vi "Squareness_2.vi"() -> ()   [LabVIEW 2020]
uses:
  Support/Controls/Cmd_Mouse Popup.ctl
  Support/Controls/Clst_Initialize Input.ctl
  Support/Controls/Cmd_Var Data IO.ctl
  Support/Controls/Cmd_STD select.ctl
  Variables/Global_Cal Info.vi
  Variables/Global_Cal STD.vi
  <vilib>/express/express arith-compare/Formula/XNode/ExpressFormulaBlockNode.xnode
panel:
  out "기준기분해능 (μm)":string
  in  "기준기 설정":string(combo)
  out "직각도":string[][](table) caption="직각도 (μm/m)"
  out "단위":string
  out "최고점":string
  out "최저점":string
  in  "Spec 변경":bool
  in  "Random":bool
  out "Spec":string[][](table)
  out "제목":string
  out "에러 출력":errorcluster
  out "Condition":string[][](table) caption="2. 직선성 시험"
  in  "Measured":string[][](table) caption="기준기 지시값 (μm)"
  out "Load?":bool
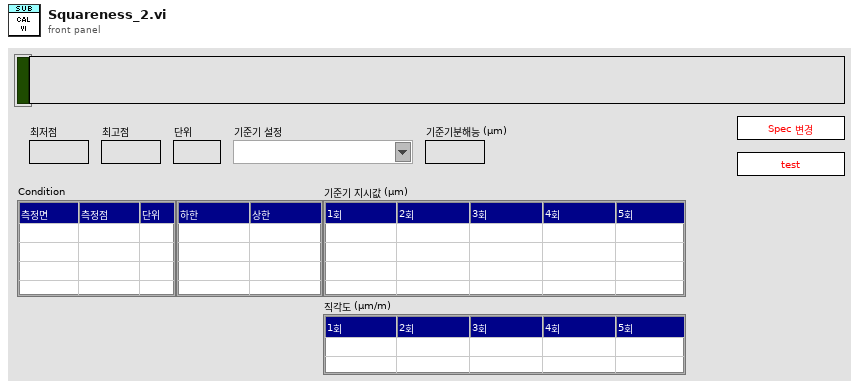
[diagram p1: front panel]
types:
  T1 = typedef "Cmd_Mouse Popup.ctl" = enum16{"활성화", "메뉴선택"}
  T2 = cluster{"Shift":bool, "Ctrl":bool, "Alt":bool, "Cmd":bool, "Opt":bool}
  T3 = typedef "Clst_Initialize Input.ctl" = cluster{"Initialize 1":cluster{"Condition":refnum<vi>[], "Spec":refnum<vi>[], "Measured":refnum<vi>[], "Resolution":refnum<vi>[], "Func_ext":string, "제목":refnum<vi>, "Measured_ADJ":refnum<vi>[]}, "Initialize 2":cluster{"문자열":refnum<vi>[], "콤보박스":refnum<vi>[], "링":refnum<vi>[], "열거형":refnum<vi>[], "테이블":refnum<vi>[], "여러열":refnum<vi>[], "디지털(DBL)":refnum<vi>[], "3D string":refnum<vi>[], "ctrl":refnum<vi>[], "boolean":refnum<vi>[]}}
  T4 = typedef "Cmd_Var Data IO.ctl" = enum16{"Condition", "Condition Default", "Condition_Temp", "Resolution", "Resolution Default", "Resolution Old", "Spec", "Spec Default", "Spec Old", "Spec Temp", "Result", "Result2", "Result3", "Result_Temp", "Result_ADJ", "Result_ADJ2", "STD1", "STD2", "STD3", "STD4", "STD5", "STD Temp", "CMC", "CMC Default"}
  T5 = typedef "Cmd_STD select.ctl" = enum16{"기본", "DMM", "Electronic Micrometer", "Fine Angle Generator", "Measuring Projector", "Precision Square", "Power Supply", "Ring Gauge", "Straight Edge", "Thermo-Hygrometer", "Calibrator"}
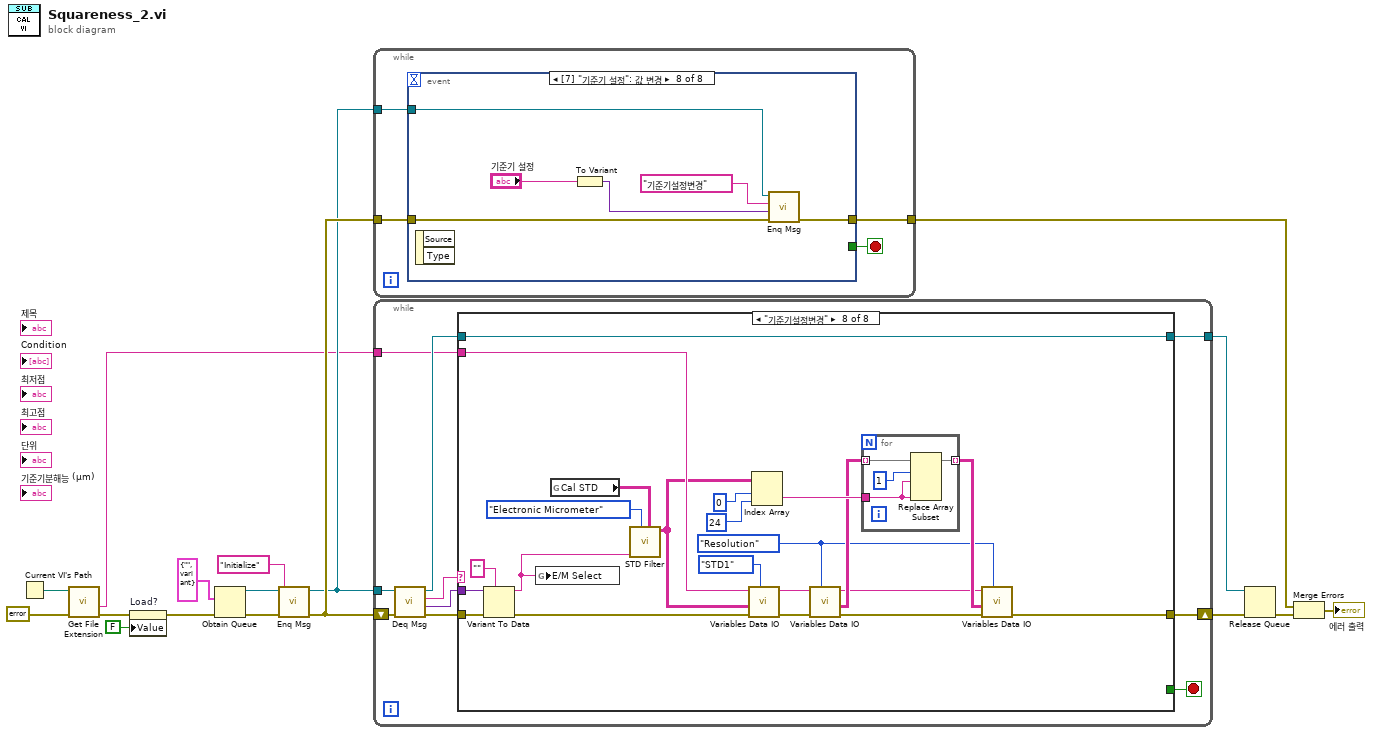
[diagram p0: block diagram]
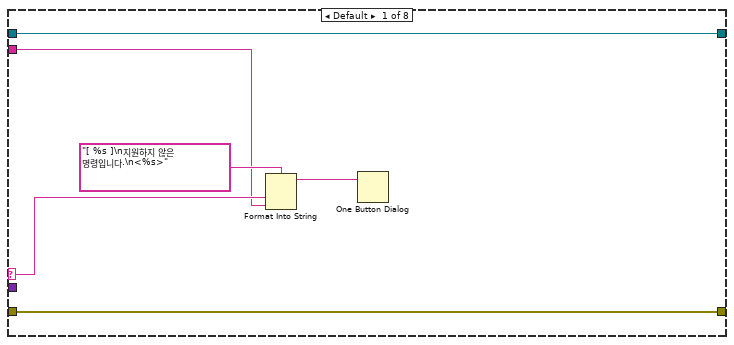
[diagram p2: hidden frame]
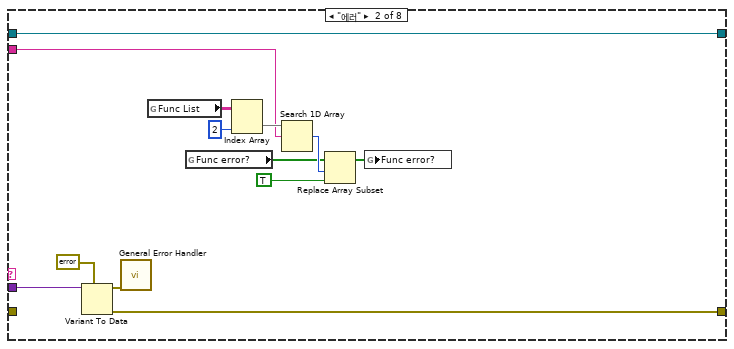
[diagram p3: hidden frame]
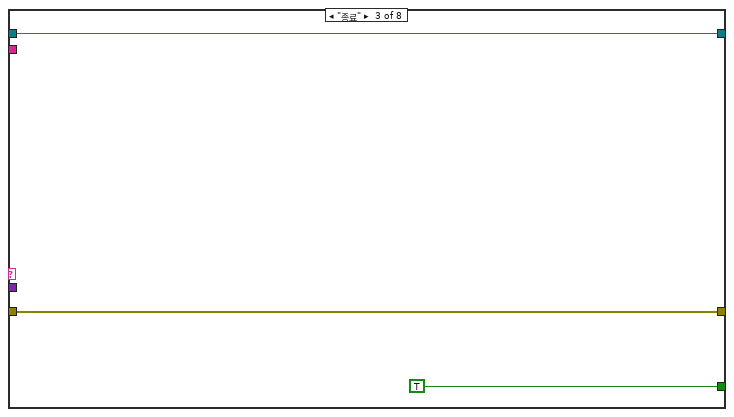
[diagram p4: hidden frame]
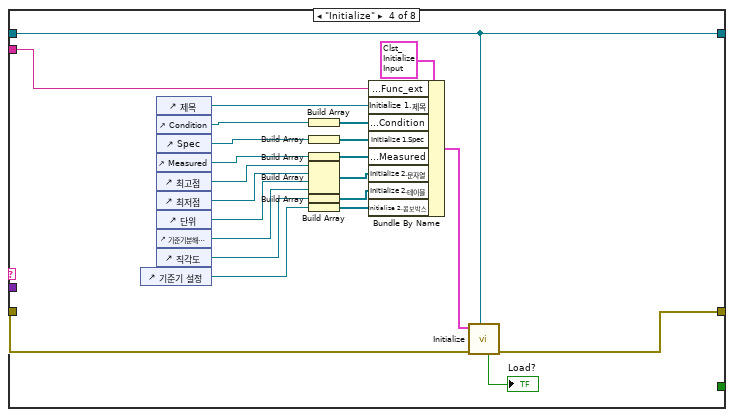
[diagram p5: hidden frame]
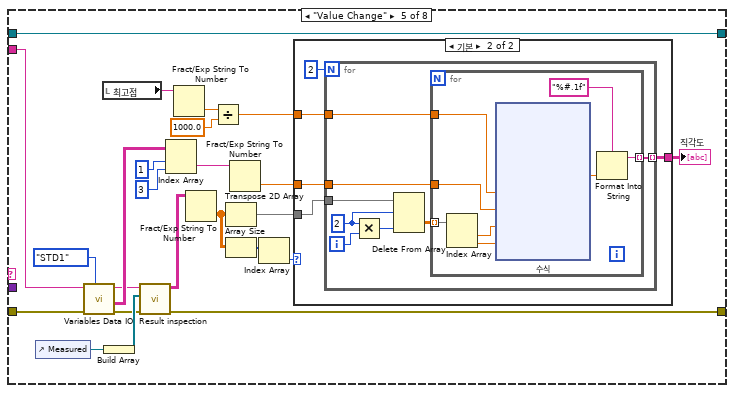
[diagram p6: hidden frame]
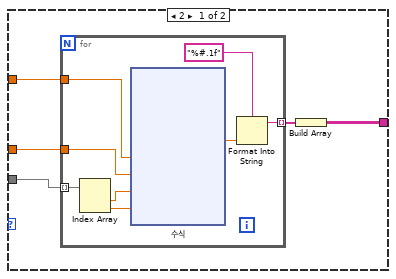
[diagram p7: hidden frame]
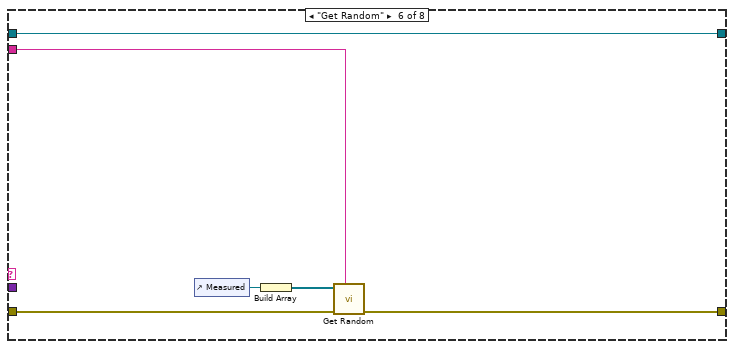
[diagram p8: hidden frame]
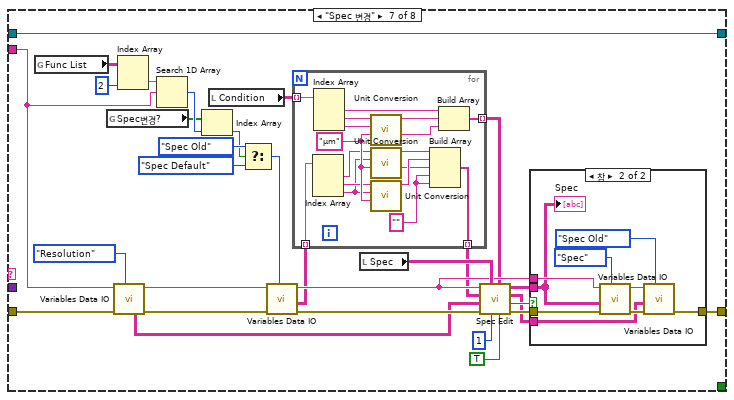
[diagram p9: hidden frame]
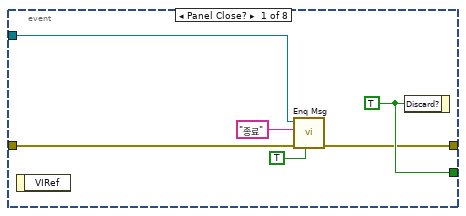
[diagram p11: hidden frame]
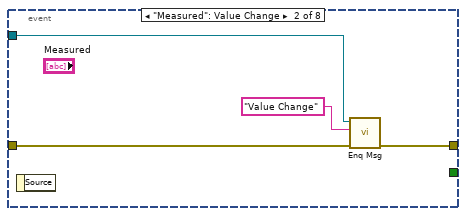
[diagram p12: hidden frame]
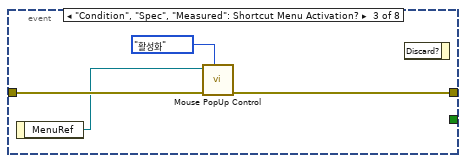
[diagram p13: hidden frame]
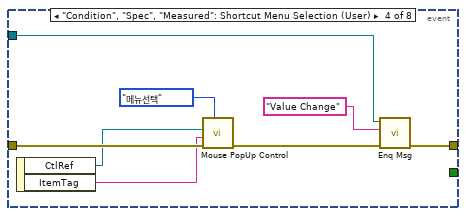
[diagram p14: hidden frame]
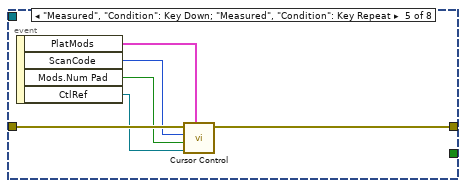
[diagram p15: hidden frame]
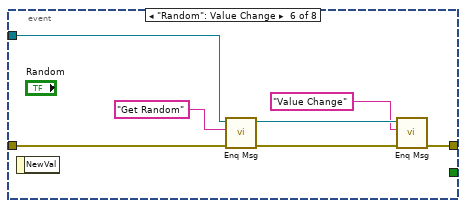
[diagram p16: hidden frame]
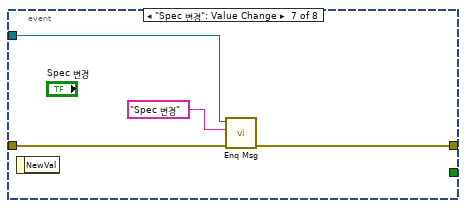
[diagram p17: hidden frame]
diagram:
  n1 = Current VI's Path() -> (path=w5:path)
  n2 = call <vilib>:"Get File Extension.vi"("error in (no error)"=errorcluster {"status"=FALSE, "code"=0, "source"=""} ("에러 상수"), "file"=w5) -> ("error out"=w3:errorcluster, "filename without extension"=w4:string)  [unwired: 5 in, 3 out]
  n3 = property on="Load?" class="Bool (엄격한)"(error in=w3, "Value"=FALSE ("Load?")) -> (error out=w2:errorcluster)  [unwired: 1 in, 1 out]
  n4 = Obtain Queue(element data type=cluster{"메세지":string, "값":variant} {"메세지"="", "값"=variant} ("Message Cluster"), error in (no error)=w2) -> (queue out=w14:refnum<queue>, error out=w16:errorcluster)  [unwired: 3 in, 1 out]
  n5 = call "Enq Msg.vi"("에러 입력(에러 없음)"=w16, "메세지"="Initialize", "큐 입력"=w14) -> ("에러 출력"=w15:errorcluster, "큐 출력"=w12:refnum<queue>)  [unwired: 7 in]
  n6 = while {
    tunnel: w15 -> [w19]
    tunnel: w12 -> [w20]
    tunnel: [w18] -> w9
    stop <- w21 stop-if-true
    n7 = event shown="[7] \"기준기 설정\": 값 변경" {
      selector: _ -> [_ _ _ _ _ _ _ _]
      dyn-events: _ -> [_ _ _ _ _ _ _ _]
      timeout: _ -> [_ _ _ _ _ _ _ _]
      tunnel: [w27 _ _ _ _ _ _ _] -> w21
      tunnel: w20 -> [w25 w31 _ w36 _ w54 w58 w64]
      tunnel: w19 -> [w26 w29 w35 w43 w49 w55 w59 w65]
      tunnel: [w23 w30 w34 w37 w48 w50 w57 w63] -> w18
      event Panel Close? {
        w27 = TRUE ("버림?")
        n8 = event-data() -> ()  [unwired: 1 in, 1 out]
        n9 = call "Enq Msg.vi"("우선순위 메시지?"=TRUE, "에러 입력(에러 없음)"=w26, "메세지"="종료", "큐 입력"=w25) -> ("에러 출력"=w23:errorcluster)  [unwired: 6 in, 1 out]
        n10 = event-data("Discard?"=w27) -> ()  [unwired: 1 in, 1 out]
      }
      event "Measured": Value Change {
        n11 = event-data() -> ()  [unwired: 1 in, 1 out]
        n12 = call "Enq Msg.vi"("에러 입력(에러 없음)"=w29, "메세지"="Value Change", "큐 입력"=w31) -> ("에러 출력"=w30:errorcluster)  [unwired: 7 in, 1 out]
      }
      event "Condition", "Spec", "Measured": Shortcut Menu Activation? {
        n13 = event-data() -> ("MenuRef"=w33:refnum<k9>)  [unwired: 1 in]
        n14 = call "Mouse PopUp Control.vi"("type"=Cmd_Mouse_Popup."활성화", "error in"=w35, "메뉴 참조"=w33) -> ("error out"=w34:errorcluster)  [unwired: 8 in]
        n15 = event-data() -> ()  [unwired: 2 in, 1 out]
      }
      event "Condition", "Spec", "Measured": Shortcut Menu Selection (User) {
        n16 = event-data() -> ("CtlRef"=w41:refnum<vi>, "ItemTag"=w40:string)  [unwired: 1 in]
        n17 = call "Mouse PopUp Control.vi"("type"=Cmd_Mouse_Popup."메뉴선택", "error in"=w43, "아이템 태그"=w40, "Tbl 참조 번호"=w41) -> ("error out"=w38:errorcluster)  [unwired: 7 in]
        n18 = call "Enq Msg.vi"("에러 입력(에러 없음)"=w38, "메세지"="Value Change", "큐 입력"=w36) -> ("에러 출력"=w37:errorcluster)  [unwired: 7 in, 1 out]
      }
      event "Measured", "Condition": Key Down; "Measured", "Condition": Key Repeat {
        n19 = event-data() -> ("PlatMods"=w44:T2, "ScanCode"=w47:i16, "Mods.Num Pad"=w46:bool, "CtlRef"=w45:refnum<vi>)  [unwired: 1 in]
        n20 = call "Cursor Control.vi"("플랫폼 조합키"=w44, "참조"=w45, "Num Pad"=w46, "ScanCode"=w47, "error in"=w49) -> ("error out"=w48:errorcluster)  [unwired: 5 in, 1 out]
      }
      event "Random": Value Change {
        n21 = event-data() -> ()  [unwired: 1 in, 1 out]
        n22 = call "Enq Msg.vi"("에러 입력(에러 없음)"=w55, "메세지"="Get Random", "큐 입력"=w54) -> ("에러 출력"=w53:errorcluster, "큐 출력"=w52:refnum<queue>)  [unwired: 7 in]
        n23 = call "Enq Msg.vi"("에러 입력(에러 없음)"=w53, "메세지"="Value Change", "큐 입력"=w52) -> ("에러 출력"=w50:errorcluster)  [unwired: 7 in, 1 out]
      }
      event "Spec 변경": Value Change {
        n24 = event-data() -> ()  [unwired: 1 in, 1 out]
        n25 = call "Enq Msg.vi"("에러 입력(에러 없음)"=w59, "메세지"="Spec 변경", "큐 입력"=w58) -> ("에러 출력"=w57:errorcluster)  [unwired: 7 in, 1 out]
      }
      event "기준기 설정": Value Change {
        n26 = event-data() -> ()  [unwired: 1 in, 2 out]
        n27 = To Variant(anything="기준기 설정") -> (Variant=w61:variant)
        n28 = call "Enq Msg.vi"("에러 입력(에러 없음)"=w65, "값"=w61, "메세지"="기준기설정변경", "큐 입력"=w64) -> ("에러 출력"=w63:errorcluster)  [unwired: 6 in, 1 out]
      }
    }
  }
  n29 = while {
    shift-right: [w76] -> w11
    shift-left: w15 -> [w75]
    tunnel: w12 -> [w73]
    tunnel: [w68] -> w10
    tunnel: w4 -> [w67]
    stop <- w69 stop-if-true
    n30 = call "Deq Msg.vi"("에러 입력(에러 없음)"=w75, "큐 입력"=w73) -> ("에러 출력"=w74:errorcluster, "값"=w70:variant, "메세지"=w72:string, "큐 출력"=w71:refnum<queue>)  [unwired: 6 in]
    n31 = case shown="\"기준기설정변경\"" w72 {
      selector: w72 -> [w78 _ _ _ _ _ _ _]
      tunnel: w74 -> [w82 _ w98 w121 w128 w209 w236 w285]
      tunnel: [w82 w92 w98 w108 w125 w210 w239 w271] -> w76
      tunnel: w71 -> [w81 w91 w96 w109 w145 w213 w243 w292]
      tunnel: w70 -> [_ w93 _ _ _ _ _ w284]
      tunnel: [_ _ TRUE ("버림?") _ _ _ _ _] -> w69
      tunnel: [w81 w91 w96 w109 w145 w213 w243 w292] -> w68
      tunnel: w67 -> [w77 w83 _ w110 w136 w208 w223 w283]
      frame Default {
        n32 = Format Into String(format string="[ %s ]\n지원하지 않은 명령입니다.\n<%s>" ("메시지"), w78, w77) -> (resulting string=w79:string)  [unwired: 2 in, 1 out]
        n33 = One Button Dialog(message=w79) -> ()  [unwired: 1 in, 1 out]
      }
      frame "에러" {
        n34 = Variant To Data(type=errorcluster {"status"=FALSE, "code"=0, "source"=""} ("에러 출력"), Variant=w93) -> (data=w95:errorcluster, error out=w92:errorcluster)  [unwired: 1 in]
        n35 = call <vilib>:"General Error Handler.vi"("error in (no error)"=w95) -> ()  [unwired: 10 in, 5 out]
        n36 = global read "Global_Cal Info.vi" "Func List"() -> (w85:string[][])
        n37 = global read "Global_Cal Info.vi" "Func error?"() -> (w88:bool[])
        n38 = Index Array(array=w85, index (col)=2 ("비활성화된 인덱스 (열)")) -> (element=w86:string[])  [unwired: 1 in]
        n39 = Search 1D Array(1D array=w86, element=w83) -> (index of element=w89:i32)  [unwired: 1 in]
        n40 = Replace Array Subset(array=w88, new element=TRUE ("새 원소/부분배열"), index=w89) -> (w90:bool[])
        n41 = global write "Global_Cal Info.vi" "Func error?"(w90) -> ()
      }
      frame "종료" {
      }
      frame "Initialize" {
        n42 = control-ref of="기준기 설정"() -> (w100:refnum<vi>)
        n43 = control-ref of="제목"() -> (w113:refnum<vi>)
        n44 = control-ref of="Condition"() -> (w118:refnum<vi>)
        n45 = control-ref of="Spec"() -> (w112:refnum<vi>)
        n46 = control-ref of="Measured"() -> (w115:refnum<vi>)
        n47 = control-ref of="최고점"() -> (w106:refnum<vi>)
        n48 = control-ref of="최저점"() -> (w105:refnum<vi>)
        n49 = control-ref of="단위"() -> (w104:refnum<vi>)
        n50 = control-ref of="기준기분해능 (μm)"() -> (w99:refnum<vi>)
        n51 = control-ref of="직각도"() -> (w103:refnum<vi>)
        n52 = Build Array(w118) -> (w117:refnum<vi>[])
        n53 = Build Array(w112) -> (w111:refnum<vi>[])
        n54 = Build Array(w115) -> (w116:refnum<vi>[])
        n55 = Build Array(w106, w105, w104, w99) -> (w114:refnum<vi>[])
        n56 = Build Array(w103) -> (w102:refnum<vi>[])
        n57 = Build Array(w100) -> (w101:refnum<vi>[])
        n58 = Bundle By Name(cluster=T3 {"Initialize 1"={"Condition"=[], "Spec"=[], "Measured"=[], "Resolution"=[], "Func_ext"="", "제목"=refnum, "Measured_ADJ"=[]}, "Initialize 2"={"문자열"=[], "콤보박스"=[], "링"=[], "열거형"=[], "테이블"=[], "여러열"=[], "디지털(DBL)"=[], "3D string"=[], "ctrl"=[], "boolean"=[]}} ("입력 클러스터"), "Initialize 1.Func_ext"=w110, "Initialize 1.제목"=w113, "Initialize 1.Condition"=w117, "Initialize 1.Spec"=w111, "Initialize 1.Measured"=w116, "Initialize 2.문자열"=w114, "Initialize 2.테이블"=w102, "Initialize 2.콤보박스"=w101) -> (w119:T3)
        n59 = call "Initialize.vi"("큐 입력"=w109, "error in"=w121, "입력 클러스터"=w119) -> ("error out"=w108:errorcluster, "Load?"=→"Load?":bool)  [unwired: 5 in, 2 out]
      }
      frame "Value Change" {
        n60 = control-ref of="Measured"() -> (w144:refnum<vi>)
        n61 = call "Variables Data IO.vi"("Select"=Cmd_Var_Data_IO."STD1", "error in"=w128, "Func_ext"=w136) -> ("error out"=w126:errorcluster, "Data Out"=w134:string[][], "Func_ext Out"=w127:string)  [unwired: 6 in]
        n62 = local read "최고점"() -> (w140:string)
        n63 = Build Array(w144) -> (w143:refnum<vi>[])
        n64 = call "Result inspection.vi"("error in"=w126, "Ref. Data (Inspection)"=w143, "Func ext"=w127) -> ("error out"=w125:errorcluster, "Data (spec 적용)"=w142:string[][])  [unwired: 5 in, 2 out]
        n65 = Index Array(array=w134, index (row)=1 ("인덱스 (행)"), index (col)=3 ("비활성화된 인덱스 (열)")) -> (element=w131:string)
        n66 = Fract/Exp String To Number(string=w140) -> (number=w139:dbl)  [unwired: 3 in, 1 out]
        n67 = Fract/Exp String To Number(string=w142) -> (number=w124:dbl[][])  [unwired: 3 in, 1 out]
        n68 = Divide(x=w139, y=1000.0) -> (x/y=w137:dbl)
        n69 = Transpose 2D Array(2D array=w124) -> (transposed array=w141:dbl[][])
        n70 = Array Size(array=w124) -> (size(s)=w123:i32[])
        n71 = Fract/Exp String To Number(string=w131) -> (number=w130:dbl)  [unwired: 3 in, 1 out]
        n72 = Index Array(array=w123) -> (element=w122:i32)  [unwired: 1 in]
        n73 = case shown="기본" w122 {
          tunnel: w141 -> [w150 w177]
          tunnel: w137 -> [w149 w176]
          tunnel: w130 -> [w148 w175]
          tunnel: [w146 w173] -> w129
          frame 2 {
            n74 = for {
              tunnel: w150 -> [w158] mode=indexing
              tunnel: w149 -> [w157]
              tunnel: w148 -> [w151]
              tunnel: [w152] -> w147 mode=indexing
              n75 = Index Array(array=w158) -> (element #1=w156:dbl, element #2=w155:dbl)  [unwired: 2 in]
              n76 = xnode "수식"("l"=w157, "T"=w151, "dmin"=w156, "dmax"=w155) -> ("결과"=w154:dbl)  [unwired: 1 in, 1 out]
              n77 = Format Into String(format string="%#.1f" ("포맷 문자열"), w154) -> (resulting string=w152:string)  [unwired: 2 in, 1 out]
            }
            n78 = Build Array(w147) -> (w146:string[][])
          }
          frame Default {
            n79 = for {
              N: 2 -> [_]
              tunnel: w177 -> [w182]
              tunnel: w176 -> [w185]
              tunnel: w175 -> [w184]
              tunnel: [w183] -> w173 mode=indexing
              i -> [w181]
              w180 = 2 ("길이")
              n80 = Multiply(x=w180, y=w181) -> (x*y=w179:i32)
              n81 = Delete From Array(array=w182, length=w180, index (col)=w179) -> (deleted portion=w178:dbl[][])  [unwired: 1 in, 1 out]
              n82 = for {
                tunnel: w178 -> [w193] mode=indexing
                tunnel: w185 -> [w192]
                tunnel: w184 -> [w186]
                tunnel: [w187] -> w183 mode=indexing
                n83 = Index Array(array=w193) -> (element #1=w191:dbl, element #2=w190:dbl)  [unwired: 2 in]
                n84 = xnode "수식"("l"=w192, "T"=w186, "dmin"=w191, "dmax"=w190) -> ("결과"=w189:dbl)  [unwired: 1 in, 1 out]
                n85 = Format Into String(format string="%#.1f" ("포맷 문자열"), w189) -> (resulting string=w187:string)  [unwired: 2 in, 1 out]
              }
            }
          }
        }
        "직각도" <- w129
      }
      frame "Get Random" {
        n86 = control-ref of="Measured"() -> (w212:refnum<vi>)
        n87 = Build Array(w212) -> (w211:refnum<vi>[])
        n88 = call "Get Random.vi"("Func_Ext"=w208, "에러 입력"=w209, "Meas"=w211) -> ("에러 출력"=w210:errorcluster)  [unwired: 7 in, 1 out]
      }
      frame "Spec 변경" {
        n89 = global read "Global_Cal Info.vi" "Func List"() -> (w228:string[][])
        n90 = global read "Global_Cal Info.vi" "Spec변경?"() -> (w224:bool[])
        n91 = call "Variables Data IO.vi"("Select"=Cmd_Var_Data_IO."Resolution", "error in"=w236, "Func_ext"=w223) -> ("error out"=w221:errorcluster, "Data Out"=w219:string[][], "Func_ext Out"=w220:string)  [unwired: 6 in]
        n92 = Index Array(array=w228, index (col)=2 ("비활성화된 인덱스 (열)")) -> (element=w226:string[])  [unwired: 1 in]
        n93 = Search 1D Array(1D array=w226, element=w223) -> (index of element=w225:i32)  [unwired: 1 in]
        n94 = Index Array(array=w224, index=w225) -> (element=w229:bool)
        n95 = local read "Condition"() -> (w217:string[][])
        n96 = Select(t=Cmd_Var_Data_IO."Spec Old" ("Select"), s=w229, f=Cmd_Var_Data_IO."Spec Default" ("Select")) -> (s? t:f=w222:T4)
        n97 = call "Variables Data IO.vi"("Select"=w222, "error in"=w221, "Func_ext"=w220) -> ("error out"=w238:errorcluster, "Data Out"=w215:string[][], "Func_ext Out"=w232:string)  [unwired: 6 in]
        n98 = for {
          tunnel: w217 -> [w247] mode=indexing
          tunnel: [w248] -> w216 mode=indexing
          tunnel: w215 -> [w257] mode=indexing
          tunnel: [w250] -> w214 mode=indexing
          w249 = "" ("원소")
          w258 = "μm" ("환산단위")
          n99 = Index Array(array=w257) -> (element #1=w256:string, element #2=w255:string, element #3=w254:string)  [unwired: 3 in]
          n100 = Index Array(array=w247) -> (element #1=w246:string, element #2=w260:string, element #3=w259:string)  [unwired: 3 in]
          n101 = call "Unit Conversion.vi"("환산단위"=w258, "입력단위"=w259, "입력값"=w260) -> ("환산단위"=w244:string, "환산값 (string)"=w245:string)  [unwired: 3 in, 4 out]
          n102 = call "Unit Conversion.vi"("환산단위"=w258, "입력단위"=w254, "입력값"=w256) -> ("환산단위"=w251:string, "환산값 (string)"=w253:string)  [unwired: 3 in, 4 out]
          n103 = call "Unit Conversion.vi"("환산단위"=w258, "입력단위"=w254, "입력값"=w255) -> ("환산값 (string)"=w252:string)  [unwired: 3 in, 5 out]
          n104 = Build Array(w253, w252, w251, w249, w249) -> (w250:string[])
          n105 = Build Array(w246, w245, w244) -> (w248:string[])
        }
        n106 = local read "Spec"() -> (w233:string[][])
        n107 = call "Spec Edit.vi"("0기준?"=TRUE, "Condition"=w216, "열번호(기준값)"=1, "Spec Value"=w233, "에러 입력(에러 없음)"=w238, "Resolution"=w219, "Spec Default"=w214, "Func_ext"=w232) -> ("에러 출력"=w240:errorcluster, "변경?"=w241:bool, "Spec Default out"=w235:string[][], "Spec 출력"=w242:string[][])
        n108 = case shown="참" w241 {
          tunnel: w242 -> [_ w267]
          tunnel: w240 -> [w261 w270]
          tunnel: [w261 w265] -> w239
          tunnel: w232 -> [_ w268]
          tunnel: w235 -> [_ w263]
          frame False {
          }
          frame True {
            n109 = call "Variables Data IO.vi"("Select"=Cmd_Var_Data_IO."Spec", "error in"=w270, "Data In"=w267, "Func_ext"=w268) -> ("error out"=w266:errorcluster, "Func_ext Out"=w264:string)  [unwired: 5 in, 1 out]
            n110 = call "Variables Data IO.vi"("Select"=Cmd_Var_Data_IO."Spec Old", "error in"=w266, "Data In"=w263, "Func_ext"=w264) -> ("error out"=w265:errorcluster)  [unwired: 5 in, 2 out]
            "Spec" <- w267
          }
        }
      }
      frame "기준기설정변경" {
        w277 = Cmd_Var_Data_IO."Resolution" ("Select")
        n111 = Variant To Data(error in=w285, type="", Variant=w284) -> (data=w289:string, error out=w290:errorcluster)
        n112 = global write "Global_Cal STD.vi" "E/M Select"(w289) -> ()
        n113 = global read "Global_Cal STD.vi" "Cal STD"() -> (w288:string[][])
        n114 = call "STD Filter.vi"("Cal STD in"=w288, "STD select"=Cmd_STD_select."Electronic Micrometer", "문자열(option, STD)"=w289) -> ("DATA 출력"=w272:string[][])  [unwired: 4 in, 4 out]
        n115 = call "Variables Data IO.vi"("Select"=Cmd_Var_Data_IO."STD1", "error in"=w290, "Data In"=w272, "Func_ext"=w283) -> ("error out"=w273:errorcluster, "Func_ext Out"=w274:string)  [unwired: 5 in, 1 out]
        n116 = Index Array(array=w272, index (row)=0 ("비활성화된 인덱스 (행)"), index (col)=24 ("비활성화된 인덱스 (열)")) -> (element=w282:string)
        n117 = call "Variables Data IO.vi"("Select"=w277, "error in"=w273, "Func_ext"=w274) -> ("error out"=w275:errorcluster, "Data Out"=w278:string[][], "Func_ext Out"=w276:string)  [unwired: 6 in]
        n118 = for {
          tunnel: w278 -> [w296] mode=indexing
          tunnel: [w295] -> w279 mode=indexing
          tunnel: w282 -> [w294]
          n119 = Replace Array Subset(array=w296, new element #1=w294, index #1=1 ("인덱스"), new element #2=w294) -> (w295:string[])  [unwired: 1 in]
        }
        n120 = call "Variables Data IO.vi"("Select"=w277, "error in"=w275, "Data In"=w279, "Func_ext"=w276) -> ("error out"=w271:errorcluster)  [unwired: 5 in, 2 out]
      }
    }
  }
  n121 = Release Queue(queue=w10, error in (no error)=w11) -> (error out=w8:errorcluster)  [unwired: 1 in, 2 out]
  n122 = Merge Errors(w9, w8) -> (→"에러 출력":errorcluster)
